vi "pressure-logger-main.vi"() -> ()   [LabVIEW 2024]
uses:
  template/state-enum.ctl
  template/csv-file-logging/filepath-selection.ctl
  template/csv-file-logging/datalogging-options.ctl
  template/serial-options.ctl
  template/sensor-options.ctl
panel:
  out "Serial Port Open":bool
  out "return count":u32
  out "Bytes at Port":u32
  out "Log File Open":bool
  in  "Tab Control":enum32{"Data", "Settings"}(tab)
  out "Units":string
  out "Data":dbl
  out "Data Plot Chart":dbl(graph)
  out "Logged CSV out":string
  out "Serial msg":string
  in  "Datalogging options":T1={"data-precision"=3, "Include Date"=FALSE, "Include Timestamp"=TRUE, "Include Milliseconds"=FALSE, "sample-rate (Hz)"=4.0, "Logging Active"=TRUE}
  in  "Log Filepath Selection":T2={"Log Filepath Source"=enum."Application Relative (Auto)", "Log File Path (Manual)"=path "C:/Users/dheard/Documents/0002-labview-projects/adam-4xxx/template/data", "Log File Folder Name"="data", "log file name"="log", "Include Date in Filename"=TRUE, "Include Time in Filename"=TRUE}
  in  "Serial Port Options":T3={"COM Port (COM10)"="COM10", "baud rate (19200)"=19200, "Simulate Hardware"=FALSE} {"baud rate (19200)" max=115200 step=1200}
  in  "Sensor Options":T4={"Display Units"="PSI", "Zero Offset"=2.62, "Sensor Min"=0.0, "Sensor Max"=500.0, "Signal Min"=0.0, "Signal Max"=100.0, "Conversion Factor"=0.0}
  in  "save-settings":bool
  in  "load-settings":bool
  in  "Settings file":path
  out "Sample Rate (Hz)":dbl format="%-#3.3f"
  in  "Debug Mode":bool
  out "Loop Time (mS)":u32
  out "State:":T5
  out "error IO":errorcluster
  in  "stop":bool
  in  "start":bool
  in  "Exit":bool
  # "Pressure Logger"
  # "Live Data"
  # "Conversion Factor to\nCalculate User Units from Sensor Units"
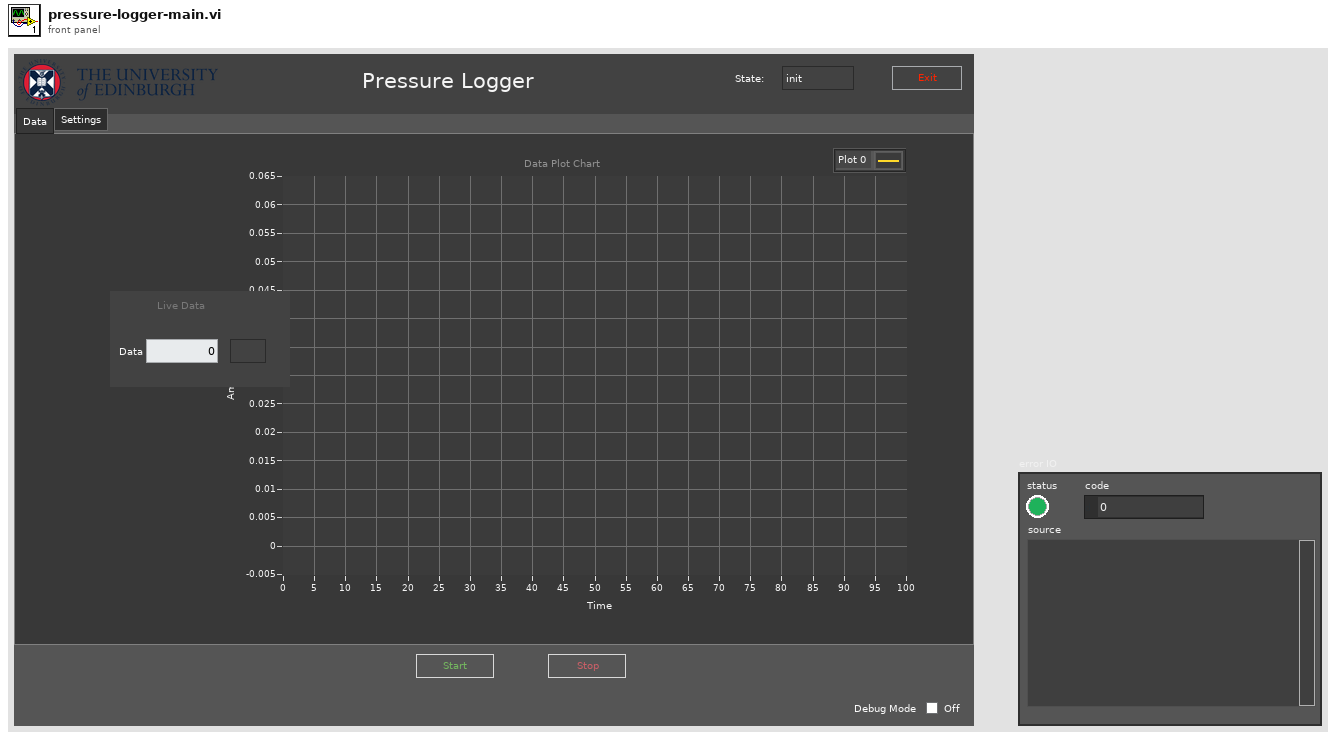
[diagram p1: front panel]
types:
  T1 = typedef "datalogging-options.ctl" = cluster{"data-precision":i32, "Include Date":bool, "Include Timestamp":bool, "Include Milliseconds":bool, "sample-rate (Hz)":dbl, "Logging Active":bool}
  T2 = typedef "filepath-selection.ctl" = cluster{"Log Filepath Source":enum16{"Application Relative (Auto)", "VI Relative (Auto)", "Complete Path (Manual)"}, "Log File Path (Manual)":path, "Log File Folder Name":string, "log file name":string, "Include Date in Filename":bool, "Include Time in Filename":bool}
  T3 = typedef "serial-options.ctl" = cluster{"COM Port (COM10)":refnum<visa-resource-name>, "baud rate (19200)":u32, "Simulate Hardware":bool}
  T4 = typedef "sensor-options.ctl" = cluster{"Display Units":string, "Zero Offset":dbl, "Sensor Min":dbl, "Sensor Max":dbl, "Signal Min":dbl, "Signal Max":dbl, "Conversion Factor":dbl}
  T5 = typedef "state-enum.ctl" = enum16{"init", "recall-settings", "save-settings", "wait", "start", "pre-run", "run", "stop", "shutdown", "exit"}
  T6 = enum8{"Enabled", "Disabled", "Disabled and Grayed Out"}
  T7 = enum16{"open", "replace", "create", "open or create", "replace or create", "replace or create with confirmation"}
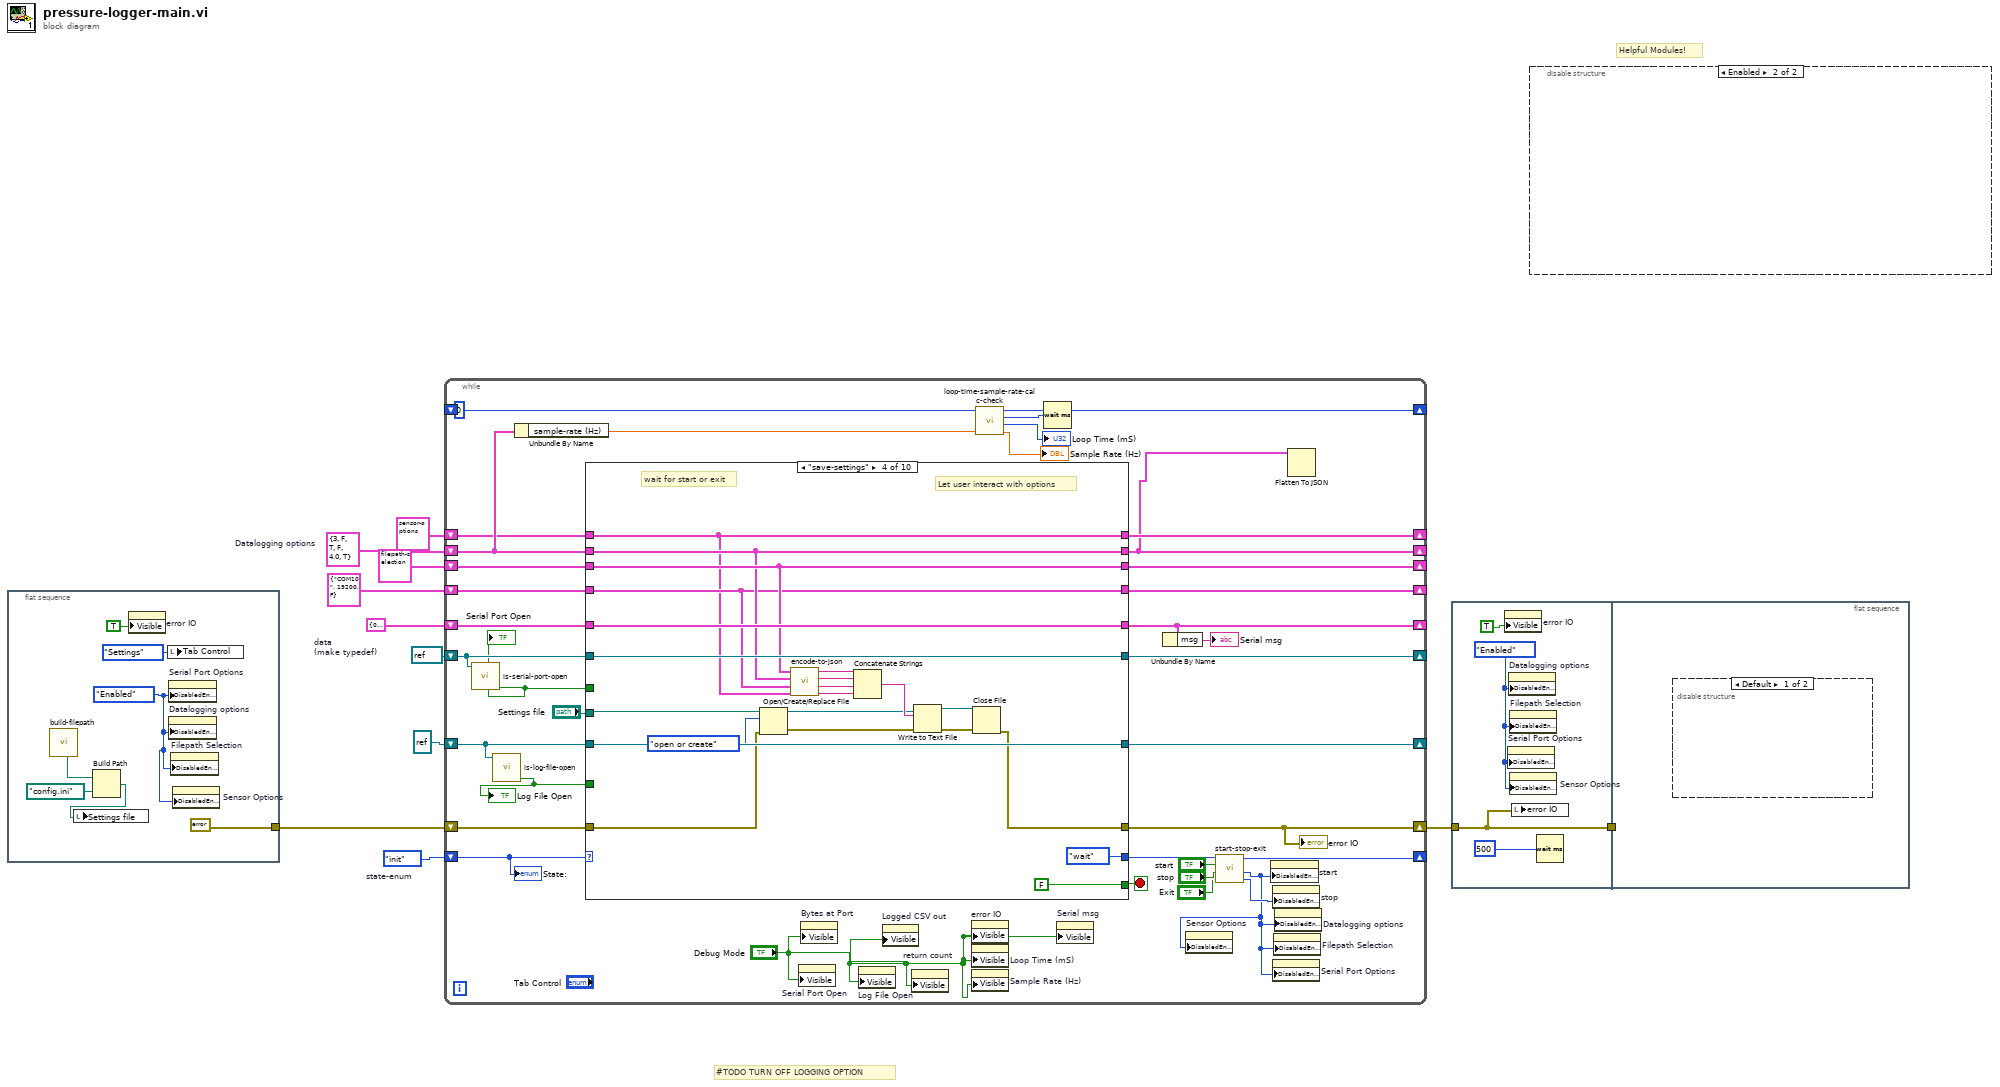
[diagram p0: block diagram]
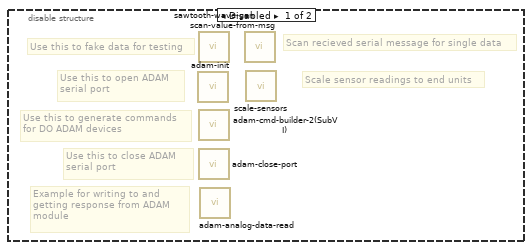
[diagram p2: hidden frame]
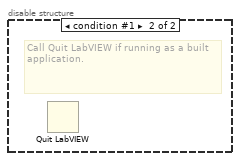
[diagram p3: hidden frame]
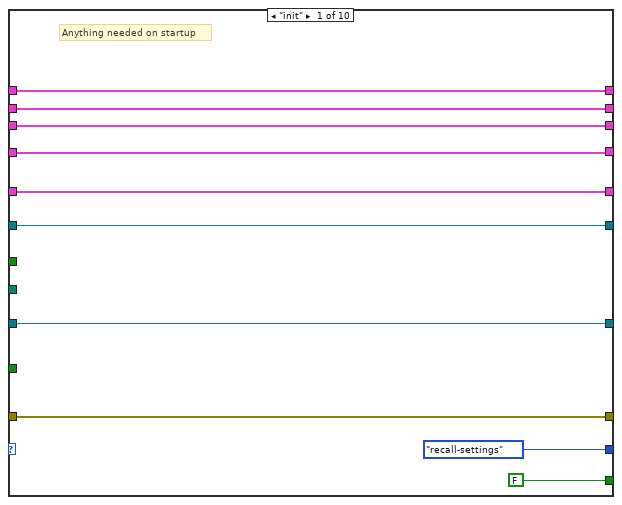
[diagram p4: hidden frame]
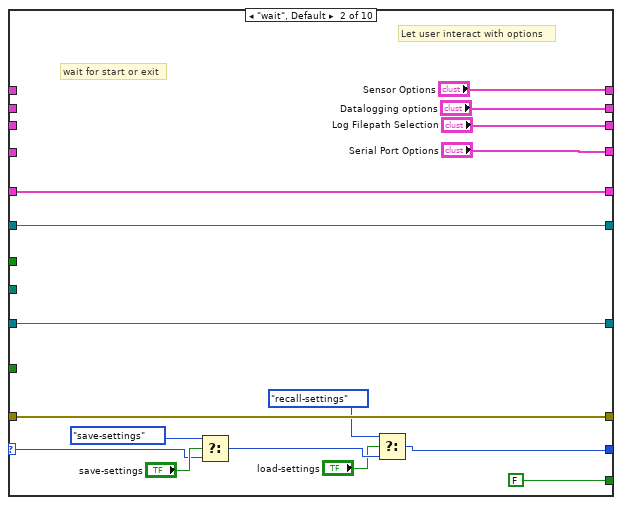
[diagram p5: hidden frame]
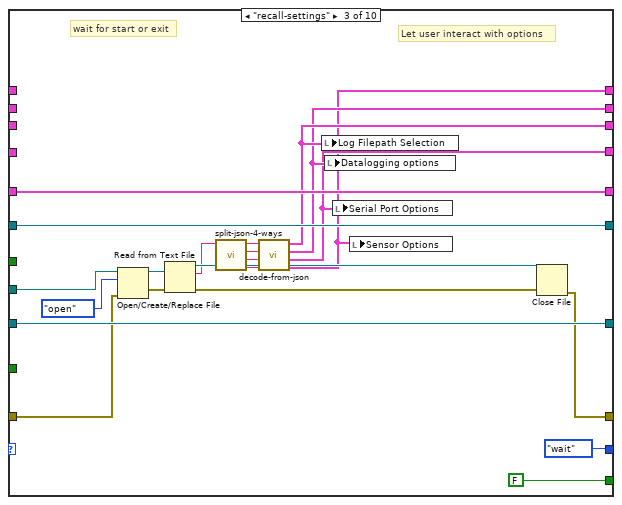
[diagram p6: hidden frame]
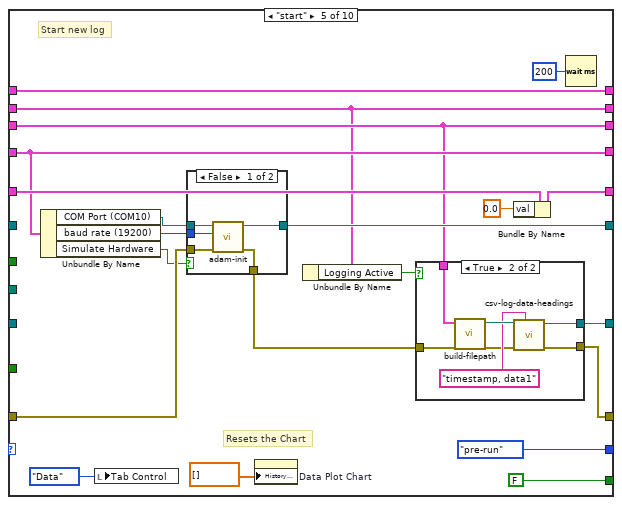
[diagram p7: hidden frame]
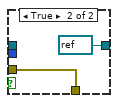
[diagram p8: hidden frame]
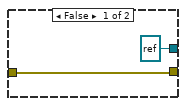
[diagram p9: hidden frame]
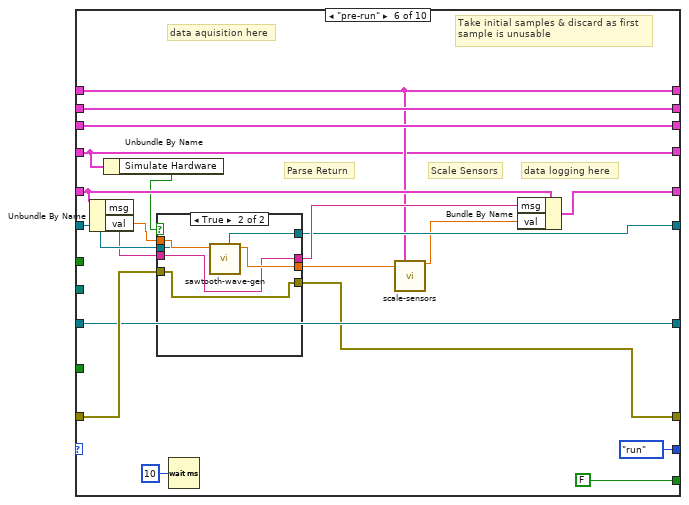
[diagram p10: hidden frame]
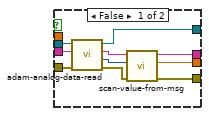
[diagram p11: hidden frame]
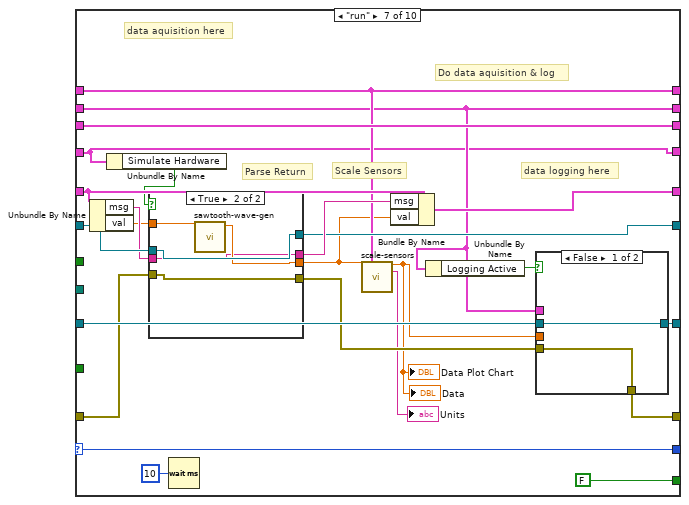
[diagram p12: hidden frame]
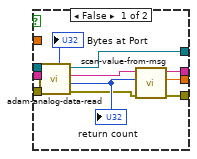
[diagram p13: hidden frame]
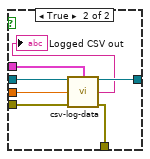
[diagram p14: hidden frame]
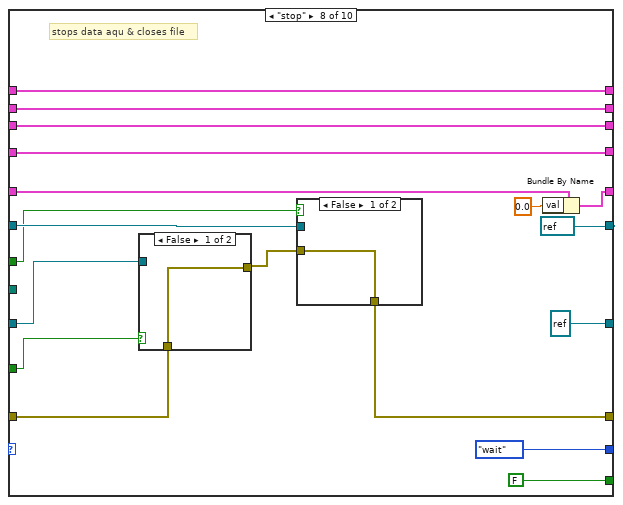
[diagram p15: hidden frame]
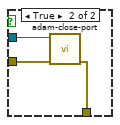
[diagram p16: hidden frame]
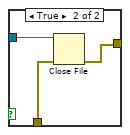
[diagram p17: hidden frame]
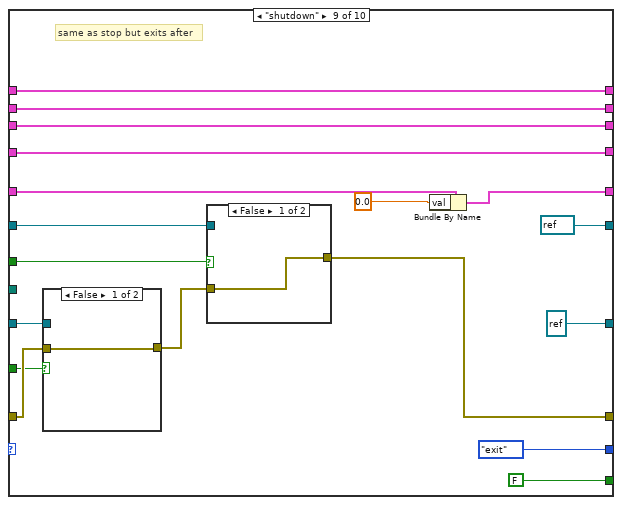
[diagram p18: hidden frame]
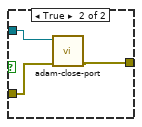
[diagram p19: hidden frame]
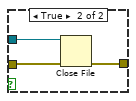
[diagram p20: hidden frame]
diagram:
  w4 = T1 {"data-precision"=3, "Include Date"=FALSE, "Include Timestamp"=TRUE, "Include Milliseconds"=FALSE, "sample-rate (Hz)"=4.0, "Logging Active"=TRUE}  # Datalogging options
  w9 = cluster{"val":dbl, "bool":bool, "msg":string} {"val"=0.0, "bool"=FALSE, "msg"=""}  # data (make typedef)
  w12 = state-enum."init"  # state-enum
  # "#TODO TURN OFF LOGGING OPTION"
  # "Helpful Modules!"
  n1 = flat-sequence {
    tunnel: [errorcluster {"status"=FALSE, "code"=0, "source"=""} ("error IO")] -> w8
    frame #0 {
      w16 = T6."Enabled" ("Disabled")
      n2 = call "build-filepath.vi"() -> ("Application Directory"=w15:path)  [unwired: 9 in, 2 out]
      n3 = Build Path(base path=w15, name or relative path=path "config.ini") -> (appended path=w13:path)
      n4 = local write "Settings file"(w13) -> ()
      n5 = property on="error IO" class="Clust (strict)"("Visible"=TRUE) -> ()  [unwired: 2 in, 2 out]
      n6 = local write "Tab Control"(enum32{"Data", "Settings"}."Settings" ("Tab Control")) -> ()
      n7 = property on="Serial Port Options" class="Clust (strict)"("DisabledEnum"=w16) -> ()  [unwired: 2 in, 2 out]
      n8 = property on="Datalogging options" class="Clust (strict)"("DisabledEnum"=w16) -> ()  [unwired: 2 in, 2 out]
      n9 = property on="Filepath Selection" class="Clust (strict)"("DisabledEnum"=w16) -> ()  [unwired: 2 in, 2 out]
      n10 = property on="Sensor Options" class="Clust (strict)"("DisabledEnum"=w16) -> ()  [unwired: 2 in, 2 out]
    }
  }
  n11 = while {
    shift-right: [w53] -> _
    shift-left: w12 -> [w55]
    shift-right: [w47] -> w10
    shift-left: w8 -> [w48]
    shift-right: [w28] -> _
    shift-left: w9 -> [w46]
    shift-right: [w43] -> _
    shift-left: u32 0 ("millisecond timer value") -> [w45]
    shift-right: [w39] -> _
    shift-left: T2 {"Log Filepath Source"=enum."Application Relative (Auto)", "Log File Path (Manual)"=path "C:/Users/dheard/Documents/0002-labview-projects/ammonia-absorbsion-rig/data", "Log File Folder Name"="data", "log file name"="log", "Include Date in Filename"=TRUE, "Include Time in Filename"=TRUE} ("Filepath Selection") -> [w38]
    shift-right: [w37] -> _
    shift-left: refnum<file> refnum ("Byte Stream File out") -> [w36]
    shift-right: [w21] -> _
    shift-left: w4 -> [w34]
    shift-right: [w31] -> _
    shift-left: T3 {"COM Port (COM10)"="COM10", "baud rate (19200)"=19200, "Simulate Hardware"=FALSE} ("Serial Port Options") -> [w32]
    shift-right: [w30] -> _
    shift-left: refnum<visa-resource-name> refnum ("VISA resource name out") -> [w29]
    shift-right: [w25] -> _
    shift-left: T4 {"Display Units"="units", "Zero Offset"=2.62, "Sensor Min"=0.0, "Sensor Max"=500.0, "Signal Min"=0.0, "Signal Max"=100.0, "Conversion Factor"=0.0} ("Sensor Options") -> [w23]
    stop <- w49 stop-if-true
    n12 = call "is-serial-port-open.vi"("VISA Refnum in"=w29) -> ("port-status"=w26:bool)  [unwired: 10 in]
    "Serial Port Open" <- w26
    n13 = call "is-log-file-open.vi"("Byte Stream File in"=w36) -> ("Log File Open"=w35:bool)  [unwired: 10 in]
    "Log File Open" <- w35
    n14 = Unbundle By Name(w34) -> ("sample-rate (Hz)"=w33:dbl)
    n15 = case shown="\"save-settings\"" w55 {
      selector: w55 -> [_ w71 _ _ _ _ w219 _ _ _]
      tunnel: [state-enum."recall-settings" w66 state-enum."wait" state-enum."wait" state-enum."pre-run" state-enum."run" w219 state-enum."wait" state-enum."exit" state-enum."exit"] -> w54
      tunnel: [FALSE FALSE FALSE FALSE FALSE FALSE FALSE FALSE FALSE TRUE] -> w49
      tunnel: [w63 w80 w92 w104 w139 w167 w214 w249 w273 w305] -> w47
      tunnel: w48 -> [w63 w80 w96 w110 w133 w176 w212 w256 w282 w305]
      tunnel: [w62 w79 w102 w124 w143 w180 w218 w259 w285 w304] -> w28
      tunnel: w46 -> [w62 w79 w102 w124 w144 w174 w210 w261 w287 w304]
      tunnel: [w60 "Log Filepath Selection" w85 w117 w129 w179 w215 w255 w281 w302] -> w39
      tunnel: w38 -> [w60 _ _ w117 w129 w179 w215 w255 w281 w302]
      tunnel: [w61 w77 w101 w123 w140 w168 w216 refnum<file> refnum ("log file Byte Stream File out") refnum<file> refnum ("log file Byte Stream File out") w303] -> w37
      tunnel: w36 -> [w61 w77 w101 w123 _ w168 w217 w258 w284 w303]
      tunnel: [w59 "Datalogging options" w84 w116 w128 w178 w202 w254 w280 w301] -> w21
      tunnel: w34 -> [w59 _ _ w116 w128 w178 w202 w254 w280 w301]
      tunnel: w35 -> [_ _ _ _ _ _ _ w247 w279 _]
      tunnel: w32 -> [w58 _ _ w115 w137 w164 w200 w253 w278 w300]
      tunnel: [w58 "Serial Port Options" w83 w115 w137 w164 w200 w253 w278 w300] -> w31
      tunnel: [w57 w74 w100 w122 w134 w171 w206 refnum<visa-resource-name> refnum ("VISA resource name out") refnum<visa-resource-name> refnum ("VISA resource name out") w299] -> w30
      tunnel: w29 -> [w57 w74 w100 w122 _ w177 w213 w252 w276 w299]
      tunnel: w26 -> [_ _ _ _ _ _ _ w246 w277 _]
      tunnel: [w56 "Sensor Options" w82 w114 w131 w170 w205 w248 w272 w298] -> w25
      tunnel: w23 -> [w56 _ _ w114 w131 w170 w205 w248 w272 w298]
      tunnel: "Settings file" -> [_ _ w98 w105 _ _ _ _ _ _]
      frame "init" {
        # "Anything needed on startup"
      }
      frame "wait", Default {
        # "Let user interact with options"
        # "wait for start or exit"
        n16 = Select(t=state-enum."save-settings", s="save-settings", f=w71) -> (s? t:f=w69:T5)
        n17 = Select(t=state-enum."recall-settings", s="load-settings", f=w69) -> (s? t:f=w66:T5)
      }
      frame "recall-settings" {
        # "Let user interact with options"
        # "wait for start or exit"
        n18 = Open/Create/Replace File(file path (use dialog)=w98, error in=w96, operation (0:open)=T7."open") -> (refnum out=w95:refnum<file>, error out=w94:errorcluster)  [unwired: 3 in, 1 out]
        n19 = Read from Text File(file (use dialog)=w95, error in=w94) -> (refnum out=w91:refnum<file>, text=w90:string, error out=w93:errorcluster)  [unwired: 2 in, 1 out]
        n20 = call "split-json-4-ways.vi"("json-string-in"=w90) -> ("sensor-json"=w86:string, "serial-json"=w87:string, "datalogging-json"=w88:string, "filepath-json"=w89:string)  [unwired: 7 in]
        n21 = call "decode-from-json.vi"("sensor-options-json"=w86, "serial-port-json"=w87, "data-logging-json"=w88, "filepath-json"=w89) -> ("Sensor Option Recall"=w82:T4, "Serial Port Recall"=w83:T3, "Datalogging Recall"=w84:T1, "Filepath Recall"=w85:T2)  [unwired: 4 in]
        n22 = local write "Log Filepath Selection"(w85) -> ()
        n23 = local write "Datalogging options"(w84) -> ()
        n24 = local write "Serial Port Options"(w83) -> ()
        n25 = local write "Sensor Options"(w82) -> ()
        n26 = Close File(refnum=w91, error in=w93) -> (error out=w92:errorcluster)  [unwired: 1 out]
      }
      frame "save-settings" {
        # "Let user interact with options"
        # "wait for start or exit"
        n27 = Open/Create/Replace File(file path (use dialog)=w105, error in=w110, operation (0:open)=T7."open or create") -> (refnum out=w109:refnum<file>, error out=w108:errorcluster)  [unwired: 3 in, 1 out]
        n28 = call "encode-to-json.vi"("Sensor Options"=w114, "Serial Port Options"=w115, "Datalogging options"=w116, "Filepath Selection"=w117) -> ("sensor-options-json"=w113:string, "serial-port-json"=w118:string, "data-logging-json"=w119:string, "filepath-json"=w120:string)  [unwired: 4 in]
        n29 = Concatenate Strings(w120, w119, w118, w113) -> (w112:string)
        n30 = Write to Text File(file (use dialog)=w109, text=w112, error in=w108) -> (refnum out=w107:refnum<file>, error out=w106:errorcluster)  [unwired: 1 in, 1 out]
        n31 = Close File(refnum=w107, error in=w106) -> (error out=w104:errorcluster)  [unwired: 1 out]
      }
      frame "start" {
        # "Start new log"
        # "Resets the Chart"
        n32 = Unbundle By Name(w137) -> ("COM Port (COM10)"=w136:refnum<visa-resource-name>, "baud rate (19200)"=w135:u32, "Simulate Hardware"=w126:bool)
        n33 = local write "Tab Control"(enum32{"Data", "Settings"}."Data" ("Tab Control")) -> ()
        n34 = case shown="False" w126 {
          tunnel: w136 -> [w151 _]
          tunnel: w135 -> [w150 _]
          tunnel: [w149 refnum<visa-resource-name> refnum ("VISA resource name out")] -> w134
          tunnel: w133 -> [w148 w152]
          tunnel: [w147 w152] -> w132
          frame False {
            n35 = call "adam-init.vi"("error in (no error)"=w148, "baud rate (19200)"=w150, "COM Port (COM10)"=w151) -> ("error out"=w147:errorcluster, "VISA resource name out"=w149:refnum<visa-resource-name>)  [unwired: 7 in]
          }
          frame True {
          }
        }
        n36 = property on="Data Plot Chart" class="WFChart (strict)"("History Data"=dbl[] []) -> ()  [unwired: 2 in, 2 out]
        n37 = Unbundle By Name(w128) -> ("Logging Active"=w127:bool)
        n38 = case shown="True" w127 {
          tunnel: [refnum<file> refnum ("Byte Stream File out") w159] -> w140
          tunnel: [w154 w158] -> w139
          tunnel: w132 -> [w154 w157]
          tunnel: w129 -> [_ w156]
          frame False {
          }
          frame True {
            n39 = call "build-filepath.vi"("Filepath Selection"=w156) -> ("appended path for log file"=w161:path)  [unwired: 8 in, 2 out]
            n40 = call "csv-log-data-headings.vi"("CSV Data Headings"="timestamp, data1", "error in (no error)"=w157, "Log File Path"=w161) -> ("error out"=w158:errorcluster, "Byte Stream File out"=w159:refnum<file>)  [unwired: 6 in, 1 out]
          }
        }
        n41 = Bundle By Name(cluster=w144, "val"=0.0 ("output")) -> (w143:cluster{"val":dbl, "bool":bool, "msg":string})
        n42 = Wait (ms)(milliseconds to wait=u32 200) -> ()  [unwired: 1 out]
      }
      frame "pre-run" {
        # "Take initial samples & discard as first\nsample is unusable"
        # "Scale Sensors"
        # "Parse Return"
        # "data logging here"
        # "data aquisition here"
        n43 = Unbundle By Name(w174) -> ("msg"=w173:string, "val"=w162:dbl)
        n44 = Unbundle By Name(w164) -> ("Simulate Hardware"=w163:bool)
        n45 = case shown="True" w163 {
          tunnel: w177 -> [w191 w192]
          tunnel: w176 -> [w190 w193]
          tunnel: w173 -> [w189 w194]
          tunnel: [w185 w194] -> w172
          tunnel: [w184 w192] -> w171
          tunnel: [w183 w195] -> w169
          tunnel: [w182 w193] -> w167
          tunnel: w162 -> [_ w196]
          frame False {
            n46 = call "adam-analog-data-read.vi"("error in (no error)"=w190, "current-buffer"=w189, "VISA Refnum in"=w191) -> ("error out"=w187:errorcluster, "return count"=w188:u32, "read buffer"=w186:string, "VISA Refnum Out"=w184:refnum<visa-resource-name>)  [unwired: 4 in, 1 out]
            n47 = call "scan-value-from-msg.vi"("error in (no error)"=w187, "msg length"=w188, "read buffer in"=w186) -> ("error out"=w182:errorcluster, "Raw Data"=w183:dbl, "read buffer out"=w185:string)  [unwired: 6 in]
          }
          frame True {
            n48 = call "sawtooth-wave-gen.vi"("current-val"=w196) -> ("output"=w195:dbl)  [unwired: 10 in]
          }
        }
        n49 = Wait (ms)(milliseconds to wait=u32 10) -> ()  [unwired: 1 out]
        n50 = call "scale-sensors.vi"("Measured Value (mV)"=w169, "Sensor Options"=w170) -> ("Calculated Value (User Specified Unit)"=w165:dbl)  [unwired: 8 in, 5 out]
        n51 = Bundle By Name(cluster=w174, "msg"=w172, "val"=w165) -> (w180:cluster{"val":dbl, "bool":bool, "msg":string})
      }
      frame "run" {
        # "Scale Sensors"
        # "Parse Return"
        # "data logging here"
        # "data aquisition here"
        # "Do data aquisition & log"
        n52 = Unbundle By Name(w210) -> ("msg"=w209:string, "val"=w198:dbl)
        n53 = Unbundle By Name(w200) -> ("Simulate Hardware"=w199:bool)
        n54 = case shown="True" w199 {
          tunnel: w213 -> [w231 w234]
          tunnel: w212 -> [w230 w236]
          tunnel: w209 -> [w228 w232]
          tunnel: [w225 w236] -> w208
          tunnel: [w223 w232] -> w207
          tunnel: [w222 w234] -> w206
          tunnel: [w221 w233] -> w197
          tunnel: w198 -> [_ w235]
          frame False {
            n55 = call "adam-analog-data-read.vi"("error in (no error)"=w230, "current-buffer"=w228, "VISA Refnum in"=w231) -> ("error out"=w226:errorcluster, "return count"=w227:u32, "read buffer"=w224:string, "VISA Refnum Out"=w222:refnum<visa-resource-name>, "Bytes at Port"=→"Bytes at Port":u32)  [unwired: 4 in]
            "return count" <- w227
            n56 = call "scan-value-from-msg.vi"("error in (no error)"=w226, "msg length"=w227, "read buffer in"=w224) -> ("error out"=w225:errorcluster, "Raw Data"=w221:dbl, "read buffer out"=w223:string)  [unwired: 6 in]
          }
          frame True {
            n57 = call "sawtooth-wave-gen.vi"("current-val"=w235) -> ("output"=w233:dbl)  [unwired: 10 in]
          }
        }
        n58 = Wait (ms)(milliseconds to wait=u32 10) -> ()  [unwired: 1 out]
        n59 = call "scale-sensors.vi"("Measured Value (mV)"=w197, "Sensor Options"=w205) -> ("Calculated Value (User Specified Unit)"=w204:dbl, "Display Units"=→"Units":string)  [unwired: 8 in, 4 out]
        "Data" <- w204
        "Data Plot Chart" <- w204
        n60 = Bundle By Name(cluster=w210, "msg"=w207, "val"=w197) -> (w218:cluster{"val":dbl, "bool":bool, "msg":string})
        n61 = Unbundle By Name(w202) -> ("Logging Active"=w201:bool)
        n62 = case shown="False" w201 {
          tunnel: w217 -> [w238 w245]
          tunnel: [w238 w244] -> w216
          tunnel: [w237 w242] -> w214
          tunnel: w202 -> [_ w241]
          tunnel: w208 -> [w237 w240]
          tunnel: w204 -> [_ w239]
          frame False {
          }
          frame True {
            n63 = call "csv-log-data.vi"("log file Byte Stream File in"=w245, "Datalogging options"=w241, "Data Point In"=w239, "error in (no error)"=w240) -> ("log file Byte Stream File out"=w244:refnum<file>, "Logged CSV out"=→"Logged CSV out":string, "error out"=w242:errorcluster)  [unwired: 7 in, 2 out]
          }
        }
      }
      frame "stop" {
        # "stops data aqu & closes file"
        n64 = case shown="False" w247 {
          tunnel: w258 -> [_ w271]
          tunnel: w256 -> [w268 w270]
          tunnel: [w268 w269] -> w250
          frame False {
          }
          frame True {
            n65 = Close File(refnum=w271, error in=w270) -> (error out=w269:errorcluster)  [unwired: 1 out]
          }
        }
        n66 = case shown="False" w246 {
          tunnel: w252 -> [_ w267]
          tunnel: w250 -> [w264 w266]
          tunnel: [w264 w265] -> w249
          frame False {
          }
          frame True {
            n67 = call "adam-close-port.vi"("error in (no error)"=w266, "VISA Refnum in"=w267) -> ("error out"=w265:errorcluster)  [unwired: 9 in]
          }
        }
        n68 = Bundle By Name(cluster=w261, "val"=0.0 ("output")) -> (w259:cluster{"val":dbl, "bool":bool, "msg":string})
      }
      frame "shutdown" {
        # "same as stop but exits after"
        n69 = case shown="False" w279 {
          tunnel: w284 -> [_ w297]
          tunnel: w282 -> [w294 w296]
          tunnel: [w294 w295] -> w274
          frame False {
          }
          frame True {
            n70 = Close File(refnum=w297, error in=w296) -> (error out=w295:errorcluster)  [unwired: 1 out]
          }
        }
        n71 = case shown="False" w277 {
          tunnel: w276 -> [_ w293]
          tunnel: w274 -> [w290 w292]
          tunnel: [w290 w291] -> w273
          frame False {
          }
          frame True {
            n72 = call "adam-close-port.vi"("error in (no error)"=w292, "VISA Refnum in"=w293) -> ("error out"=w291:errorcluster)  [unwired: 9 in]
          }
        }
        n73 = Bundle By Name(cluster=w287, "val"=0.0 ("output")) -> (w285:cluster{"val":dbl, "bool":bool, "msg":string})
      }
      frame "exit" {
        # "Exit safely"
      }
    }
    "error IO" <- w47
    n74 = property on="Serial Port Open" class="Bool (strict)"("Visible"="Debug Mode") -> ()  [unwired: 2 in, 2 out]
    n75 = property on="Bytes at Port" class="DigNum (strict)"("Visible"="Debug Mode") -> ()  [unwired: 2 in, 2 out]
    n76 = property on="Log File Open" class="Bool (strict)"("Visible"="Debug Mode") -> ()  [unwired: 2 in, 2 out]
    n77 = property on="Logged CSV out" class="Str"("Visible"="Debug Mode") -> ()  [unwired: 2 in, 2 out]
    n78 = property on="return count" class="DigNum (strict)"("Visible"="Debug Mode") -> ()  [unwired: 2 in, 2 out]
    n79 = property on="error IO" class="Clust (strict)"("Visible"="Debug Mode") -> ()  [unwired: 2 in, 2 out]
    n80 = property on="Loop Time (mS)" class="DigNum (strict)"("Visible"="Debug Mode") -> ()  [unwired: 2 in, 2 out]
    n81 = property on="Sample Rate (Hz)" class="DigNum (strict)"("Visible"="Debug Mode") -> ()  [unwired: 2 in, 2 out]
    n82 = call "loop-time-sample-rate-calc-check.vi"("sample-rate-Hz"=w33, "millisecond timer value in"=w45) -> ("Loop Hz"=→"Sample Rate (Hz)":dbl, "Loop Time (mS)"=→"Loop Time (mS)":u32, "sample-rate-delay-mS"=w40:u32, "millisecond timer value out"=w43:u32)  [unwired: 6 in]
    n83 = Wait (ms)(milliseconds to wait=w40) -> ()  [unwired: 1 out]
    n84 = property on="Serial msg" class="Str"("Visible"="Debug Mode") -> ()  [unwired: 2 in, 2 out]
    n85 = Unbundle By Name(w28) -> ("msg"=→"Serial msg":string)
    n86 = call "start-stop-exit.vi"("Exit"="Exit", "stop"="stop", "start"="start", "current-state"=w54) -> ("stop-enable"=w44:T6, "start-enable"=w24:T6, "new-state"=w53:T5)  [unwired: 5 in]
    n87 = property on="Sensor Options" class="Clust (strict)"("DisabledEnum"=w24) -> ()  [unwired: 2 in, 2 out]
    n88 = property on="start" class="Bool"("DisabledEnum"=w24) -> ()  [unwired: 2 in, 2 out]
    n89 = property on="stop" class="Bool"("DisabledEnum"=w44) -> ()  [unwired: 2 in, 2 out]
    n90 = property on="Serial Port Options" class="Clust (strict)"("DisabledEnum"=w24) -> ()  [unwired: 2 in, 2 out]
    n91 = property on="Filepath Selection" class="Clust (strict)"("DisabledEnum"=w24) -> ()  [unwired: 2 in, 2 out]
    n92 = property on="Datalogging options" class="Clust (strict)"("DisabledEnum"=w24) -> ()  [unwired: 2 in, 2 out]
    n93 = Flatten To JSON(anything=w21) -> ()  [unwired: 2 in, 2 out]
    "State:" <- w55
  }
  n94 = flat-sequence {
    tunnel: [w309] -> w11
    tunnel: w10 -> [w309]
    tunnel: w11 -> [_]
    frame #0 {
      w308 = T6."Enabled" ("Disabled")
      n95 = property on="error IO" class="Clust (strict)"("Visible"=TRUE) -> ()  [unwired: 2 in, 2 out]
      n96 = property on="Serial Port Options" class="Clust (strict)"("DisabledEnum"=w308) -> ()  [unwired: 2 in, 2 out]
      n97 = property on="Datalogging options" class="Clust (strict)"("DisabledEnum"=w308) -> ()  [unwired: 2 in, 2 out]
      n98 = property on="Filepath Selection" class="Clust (strict)"("DisabledEnum"=w308) -> ()  [unwired: 2 in, 2 out]
      n99 = property on="Sensor Options" class="Clust (strict)"("DisabledEnum"=w308) -> ()  [unwired: 2 in, 2 out]
      n100 = local write "error IO"(w309) -> ()
      n101 = Wait (ms)(milliseconds to wait=u32 500) -> ()  [unwired: 1 out]
    }
    frame #1 {
      n102 = disable-structure "Conditional Disable Structure" shown="Default" {
        frame condition #0 (active) {
        }
        frame condition #1 {
          # "Call Quit LabVIEW if running as a built application."
          n103 = Quit LabVIEW() -> ()  [unwired: 1 in]
        }
      }
    }
  }
  n104 = disable-structure shown="Enabled" {
    frame Disabled {
      # "Scale sensor readings to end units"
      # "Scan recieved serial message for single data"
      # "Example for writing to and\ngetting response from ADAM\nmodule"
      # "Use this to open ADAM\nserial port"
      # "Use this to close ADAM \nserial port"
      # "Use this to generate commands\nfor DO ADAM devices"
      # "Use this to fake data for testing"
      n105 = call "adam-init.vi"() -> ()  [unwired: 10 in, 2 out]
      n106 = call "sawtooth-wave-gen.vi"() -> ()  [unwired: 11 in, 1 out]
      n107 = call "adam-cmd-builder-2(SubVI).vi"() -> ()  [unwired: 6 in, 6 out]
      n108 = call "adam-close-port.vi"() -> ()  [unwired: 11 in, 1 out]
      n109 = call "adam-analog-data-read.vi"() -> ()  [unwired: 7 in, 5 out]
      n110 = call "scan-value-from-msg.vi"() -> ()  [unwired: 9 in, 3 out]
      n111 = call "scale-sensors.vi"() -> ()  [unwired: 10 in, 6 out]
    }
    frame Enabled {
    }
  }
